vi "PXI-Wait For AO Write Space.vi"(0 "Task In":refnum<k21>, 5 "Timeout (ms)":i32, 7 "Size":i32, 11 "error in (no error)":errorcluster) -> (4 "Task Out":refnum<k21>, 15 "error out":errorcluster)   [LabVIEW 2020]
uses:
  <resource>/objmgr/daqmx.rc
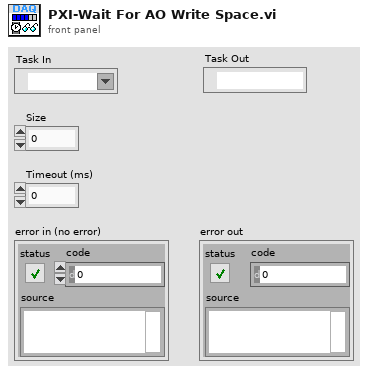
[diagram p1: front panel]
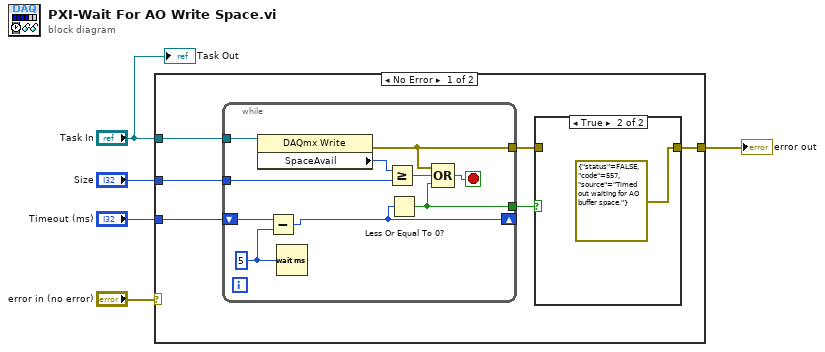
[diagram p0: block diagram]
diagram:
  n1 = case shown="No Error" "error in (no error)" {
    selector: "error in (no error)" -> [_ w24]
    tunnel: "Task In" -> [w11 _]
    tunnel: "Size" -> [w10 _]
    tunnel: "Timeout (ms)" -> [w9 _]
    tunnel: [w6 w24] -> w5
    frame No Error {
      n2 = while {
        tunnel: w11 -> [w23]
        tunnel: w10 -> [w21]
        shift-right: [w18] -> _
        shift-left: w9 -> [w20]
        tunnel: [w15] -> w8
        tunnel: [w14] -> w7
        stop <- w16 stop-if-true
        w19 = 5
        n3 = property class="DAQmx Write"(reference=w23) -> (error out=w14:errorcluster, "SpaceAvail"=w22:u32)  [unwired: 1 in, 1 out]
        n4 = Subtract(x=w20, y=w19) -> (x-y=w18:i32)
        n5 = Wait (ms)(milliseconds to wait=w19) -> ()  [unwired: 1 out]
        n6 = Greater Or Equal?(x=w22, y=w21) -> (x >= y?=w17:bool)
        n7 = Less Or Equal To 0?(x=w18) -> (x <= 0?=w15:bool)
        n8 = Compound Arithmetic op=OR(w14, w17, w15) -> (w16:bool)
      }
      n9 = case shown="True" w8 {
        tunnel: w7 -> [w12 _]
        tunnel: [w12 errorcluster {"status"=FALSE, "code"=557, "source"="Timed out waiting for AO buffer space."} ("error out 2")] -> w6
        frame False {
        }
        frame True {
        }
      }
    }
    frame Error {
    }
  }
  "error out" <- w5
  "Task Out" <- "Task In"
